vi "Meas Result Update Reading Status.vi"(4 "dvm reading":T2={"U [V]"=nan, "f [Hz]"=nan, "unc(U) [V] (k=2)"=nan, "formated rdg str"=""}, 6 "dvm ref":refnum<vi>, 8 "error in":errorcluster, 9 "sweep item":T1 {"bias" format="%#_3p"; "level" format="%#_3p"; "fs [Hz]" format="%#_5p"; "time [s]" format="%#_3p"; "f/fs" format="%#_3p"; "periods" format="%#_3f"; "f [Hz]" format="%#_5p"}, 10 "reading":T3, 11 "str ref":refnum<vi>) -> (0 "error out":errorcluster)   [LabVIEW 2020]
doc: "Updates status line with current reading data."
uses:
  bridge/Bridge Reading Data.ctl
  drivers/TWM client/Meas Proc QWTB Spectrum Data.ctl
  drivers/TWM client/TWM Phase Info.ctl
  dvm/dvm Reading.ctl
  Meas Freq Info.ctl
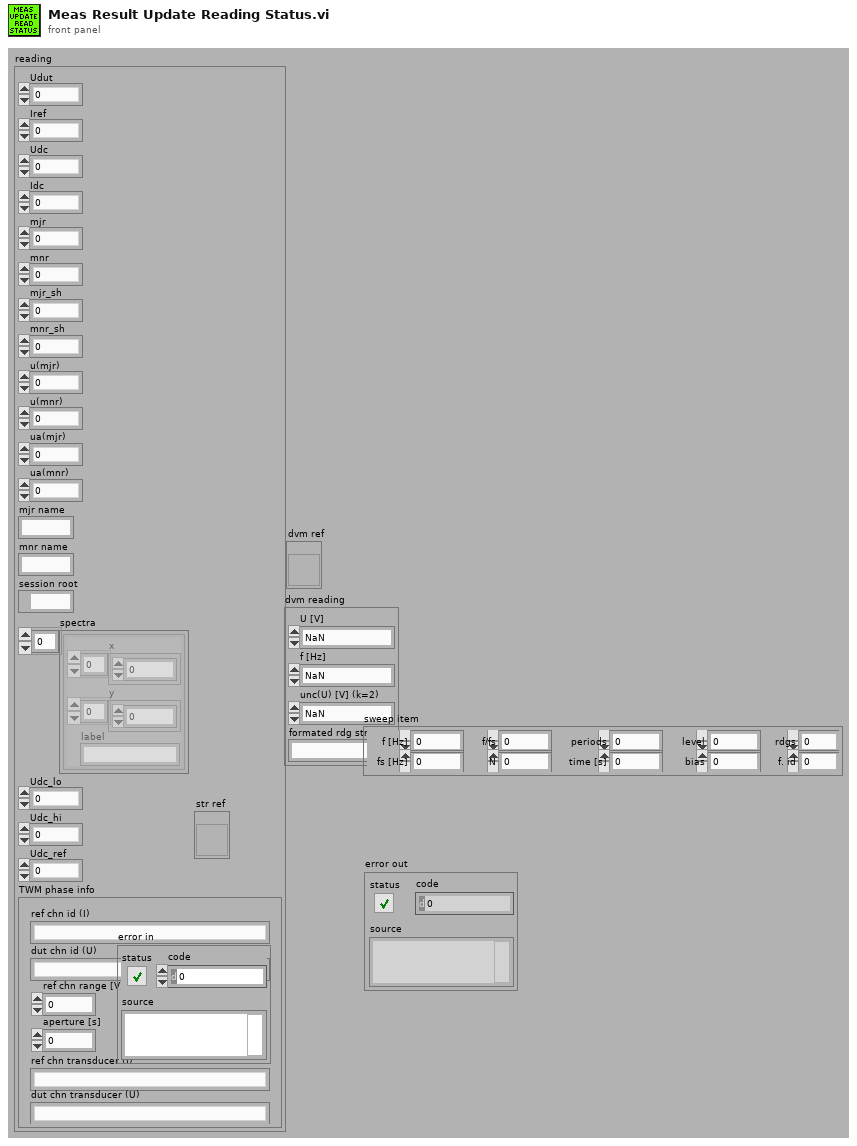
[diagram p1: front panel]
types:
  T1 = typedef "Meas Freq Info.ctl" = cluster{"f [Hz]":dbl, "periods":dbl, "f/fs":dbl, "time [s]":dbl, "fs [Hz]":dbl, "N":i32, "level":dbl, "bias":dbl, "rdgs":i32, "f. id":i32}
  T2 = typedef "dvm Reading.ctl" = cluster{"U [V]":dbl, "f [Hz]":dbl, "unc(U) [V] (k=2)":dbl, "formated rdg str":string}
  T3 = typedef "Bridge Reading Data.ctl" = cluster{"Udut":dbl, "Iref":dbl, "Udc":dbl, "Idc":dbl, "mjr":dbl, "mnr":dbl, "mjr_sh":dbl, "mnr_sh":dbl, "u(mjr)":dbl, "u(mnr)":dbl, "ua(mjr)":dbl, "ua(mnr)":dbl, "mjr name":string, "mnr name":string, "session root":path, "spectra":T4[], "Udc_lo":dbl, "Udc_hi":dbl, "Udc_ref":dbl, "TWM phase info":T5}
  T4 = typedef "Meas Proc QWTB Spectrum Data.ctl" = cluster{"x":sgl[], "y":sgl[], "label":string}
  T5 = typedef "TWM Phase Info.ctl" = cluster{"ref chn id (I)":string, "dut chn id (U)":string, "ref chn range [V]":dbl, "dut chn range [V]":dbl, "aperture [s]":dbl, "fs [Hz]":dbl, "ref chn transducer (I)":string, "dut chn transducer (U)":string}
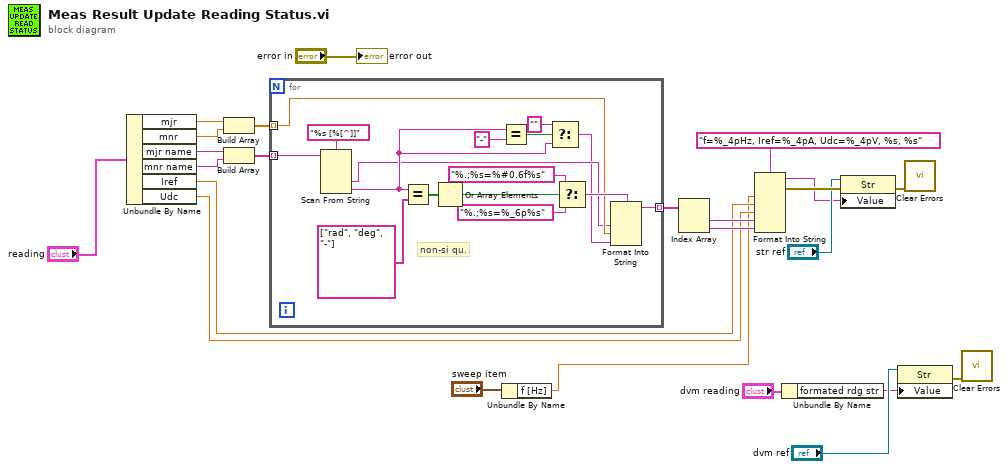
[diagram p0: block diagram]
diagram:
  n1 = Unbundle By Name("reading") -> ("mjr"=w22:dbl, "mnr"=w21:dbl, "mjr name"=w20:string, "mnr name"=w19:string, "Iref"=w13:dbl, "Udc"=w12:dbl)
  n2 = Build Array(w22, w21) -> (w18:dbl[])
  n3 = Build Array(w20, w19) -> (w17:string[])
  n4 = for {
    tunnel: w18 -> [w30] mode=indexing
    tunnel: w17 -> [w40] mode=indexing
    tunnel: [w27] -> w16 mode=indexing
    # "non-si qu."
    n5 = Scan From String(format string="%s [%[^]]", input string=w40) -> (output 1=w29:string, output 2=w33:string)  [unwired: 4 in, 3 out]
    n6 = Equal?(x=w33, y=string[] ["rad", "deg", "-"]) -> (x = y?=w37:bool[])
    n7 = Or Array Elements(Boolean array=w37) -> (logical OR=w36:bool)
    n8 = Equal?(x=w33, y="-") -> (x = y?=w34:bool)
    n9 = Select(t="", s=w34, f=w33) -> (s? t:f=w28:string)
    n10 = Select(t="%.;%s=%#0.6f%s" ("format string"), s=w36, f="%.;%s=%_6p%s" ("format string")) -> (s? t:f=w31:string)
    n11 = Format Into String(format string=w31, w29, w30, w28) -> (resulting string=w27:string)  [unwired: 2 in, 1 out]
  }
  n12 = Unbundle By Name("sweep item") -> ("f [Hz]"=w1:dbl)
  n13 = Index Array(array=w16) -> (element #1=w15:string, element #2=w14:string)  [unwired: 2 in]
  n14 = Format Into String(format string="f=%_4pHz, Iref=%_4pA, Udc=%_4pV, %s, %s", w1, w13, w12, w15, w14) -> (resulting string=w8:string, error out=w10:errorcluster)  [unwired: 2 in]
  n15 = Unbundle By Name("dvm reading") -> ("formated rdg str"=w3:string)
  n16 = property class="Str"(reference="str ref", error in=w10, "Value"=w8) -> (error out=w7:errorcluster)  [unwired: 1 out]
  n17 = property class="Str"(reference="dvm ref", "Value"=w3) -> (error out=w6:errorcluster)  [unwired: 1 in, 1 out]
  n18 = call <vilib>:"Clear Errors.vi"("error in (no error)"=w7) -> ()  [unwired: 5 in, 2 out]
  n19 = call <vilib>:"Clear Errors.vi"("error in (no error)"=w6) -> ()  [unwired: 5 in, 2 out]
  "error out" <- "error in"
